vi "Main.vi"() -> ()   [LabVIEW 2019]
uses:
  Sub VIs/State Estimator/Measurements.ctl
  Sub VIs/IMU/IMU Data.ctl
  Sub VIs/Steering Motor Encoder/Steering Motor Encoder Data.ctl
  Sub VIs/GNSS/GNSS Data.ctl
  Sub VIs/State Estimator/State Estimate.ctl
  Sub VIs/Logging/Controller Data.ctl
  Sub VIs/Drive Motor/Drive Motor Data.ctl
  Sub VIs/Steering Motor/Steering Motor Data.ctl
  Sub VIs/Logging/Log Level.ctl
  <vilib>/Platform/TimedLoop/XDataNode/timing_clust.ctl
  <vilib>/Platform/TimedLoop/XDataNode/nitl_modes.ctl
  <vilib>/Platform/TimedLoop/XDataNode/wakeup.ctl
  <vilib>/platform/TimedLoop/XDataNode/XDataNode.xnode
  <vilib>/Platform/TimedLoop/XDataNode/XDNodeRunTimeDep.lvlib
panel:
  out "Motor Controllers (Debug)":T1
  in  "Angular Speed (rad/s)":dbl
  in  "Enable Steering Motor":bool
  out "Steering Motor Enabled":bool
  out "State Estimate (Debug)":T4
  out "Measurements (Debug)":T5
  out "Abort":bool
  in  "Reset Counter":bool
  in  "Stop Button":bool
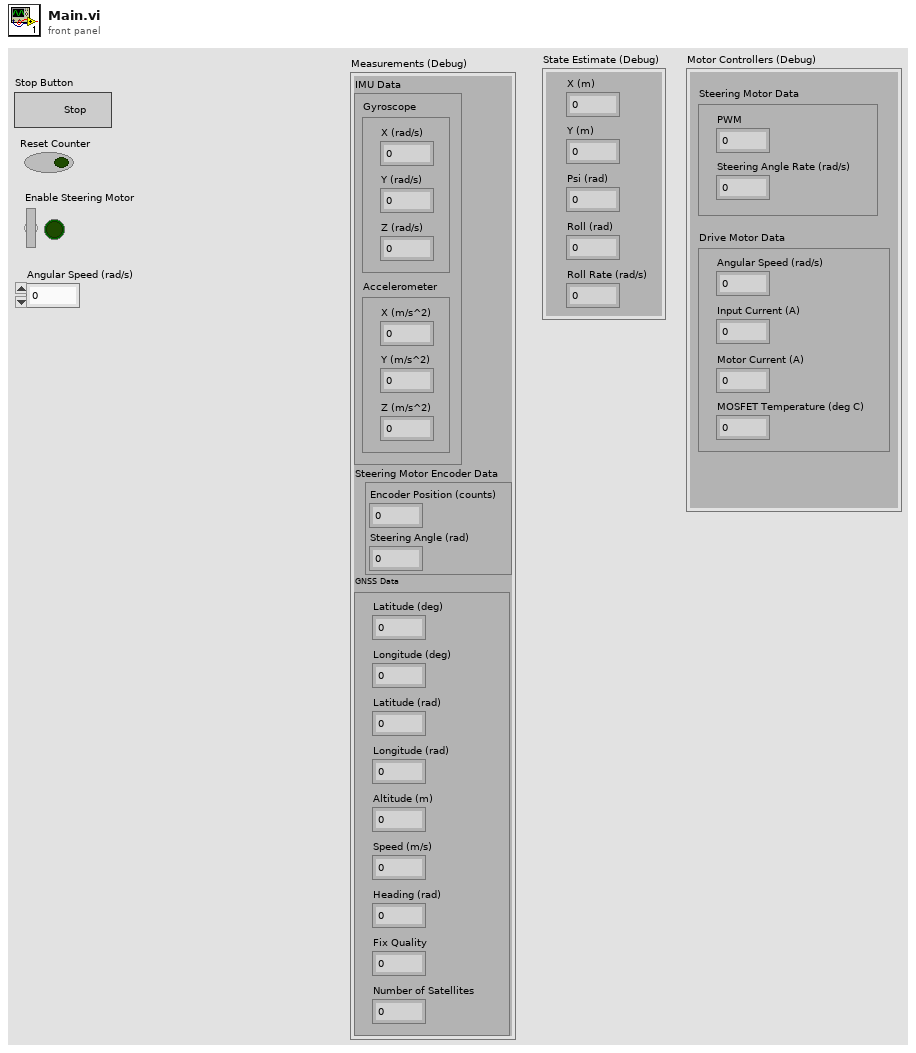
[diagram p1: front panel]
types:
  T1 = typedef "Controller Data.ctl" = cluster{"Drive Motor Data":T2, "Steering Motor Data":T3}
  T2 = typedef "Drive Motor Data.ctl" = cluster{"Angular Speed (rad/s)":dbl, "Input Current (A)":dbl, "Motor Current (A)":dbl, "MOSFET Temperature (deg C)":dbl}
  T3 = typedef "Steering Motor Data.ctl" = cluster{"PWM":dbl, "Steering Angle Rate (rad/s)":dbl}
  T4 = typedef "State Estimate.ctl" = cluster{"X (m)":dbl, "Y (m)":dbl, "Psi (rad)":dbl, "Roll (rad)":dbl, "Roll Rate (rad/s)":dbl}
  T5 = typedef "Measurements.ctl" = cluster{"IMU Data":T6, "Steering Motor Encoder Data":T7, "GNSS Data":T8}
  T6 = typedef "IMU Data.ctl" = cluster{"Gyroscope":cluster{"X (rad/s)":dbl, "Y (rad/s)":dbl, "Z (rad/s)":dbl}, "Accelerometer":cluster{"X (m/s^2)":dbl, "Y (m/s^2)":dbl, "Z (m/s^2)":dbl}}
  T7 = typedef "Steering Motor Encoder Data.ctl" = cluster{"Encoder Position (counts)":i32, "Steering Angle (rad)":dbl}
  T8 = typedef "GNSS Data.ctl" = cluster{"Latitude (rad)":dbl, "Longitude (rad)":dbl, "Altitude (m)":dbl, "Speed (m/s)":dbl, "Heading (rad)":dbl, "Fix Quality":i32, "Number of Satellites":i32, "Latitude (deg)":dbl, "Longitude (deg)":dbl}
  T9 = typedef "XDNodeRunTimeDep.lvlib/timing_clust.ctl" = cluster{"Expected End [f-1]":u64, "Actual End [f-1]":u64, "Finished Late? [f-1]":bool, "Expected End [i-1]":u64, "Actual End [i-1]":u64, "Finished Late? [i-1]":bool, "Expected Start [i]":u64, "Actual Start [i]":u64, "Expected Start [f]":u64, "Actual Start [f]":u64, "Source Name":string, "Structure Name":string, "Period":i64, "Deadline":i64, "Offset":i64, "Start":i64, "Priority":i32, "Timeout":i32, "Mode":T10, "Wakeup Reason":T11, "Error":errorcluster, "Source Type":string, "Secondary Source Type":string, "Global End Time":u64, "Global Start Time":u64, "Frame Duration":u64, "Iteration Duration":u64, "Assigned CPU":i32, "I/O Scan Engine Mode":u32}
  T10 = typedef "XDNodeRunTimeDep.lvlib/nitl_modes.ctl" = enum32{"No Change", "Process missed periods, maintain original phase", "Discard missed periods, maintain original phase", "Process missed periods, ignore original phase", "Discard missed periods, ignore original phase"}
  T11 = typedef "XDNodeRunTimeDep.lvlib/wakeup.ctl" = enum32{"Normal", "Aborted", "Asynchronous wakeup", "Timing source error", "Timed loop error", "Timeout"}
  T12 = typedef "Log Level.ctl" = enum16{"Error", "Warning", "Info"}
  T13 = typedef "Configuration.ctl" = cluster{"Accelerometer Bias":cluster{"X (m/s)":dbl, "Y (m/s)":dbl, "Z (m/s)":dbl}, "Gyroscope Bias":cluster{"X (m/s)":dbl, "Y (m/s)":dbl, "Z (m/s)":dbl}, "Steering Motor Gear Ratio":dbl, "Steering Pully Gear Ratio":dbl, "Steering Encoder CPR":dbl, "Steering Motor Max RPM":dbl, "Wheelbase (m)":dbl, "Fork Angle (rad)":dbl, "Balancing Controller":cluster{"Kp (/s)":dbl, "Kd (1)":dbl}, "Max Allowed Steering Angle (rad)":dbl, "Task Periods":cluster{"Emergency Stop (us)":i64, "IMU (us)":i64, "Steering Motor Encoder (us)":i64, "State Estimator (us)":i64, "Balancing Controller (us)":i64, "GNSS (us)":i64, "Logging (us)":i64, "Drive Motor (us)":i64}, "Drive Motor Gear Ratio":dbl, "Drive Motor UART Delay (ms)":i64}
  T14 = typedef "IMU Handle.ctl" = cluster{"I2C address":u8}
  T15 = typedef "GNSS Handle.ctl" = cluster{"VISA Resource Name":refnum<visa-resource-name>}
  T16 = typedef "Drive Motor Handle.ctl" = cluster{"VISA Resource Name":refnum<visa-resource-name>}
  T17 = typedef "Steering Motor Handle.ctl" = cluster{"Dummy":dbl}
  T18 = typedef "Log Handle.ctl" = cluster{"Data File":refnum<file>, "Event File":refnum<file>}
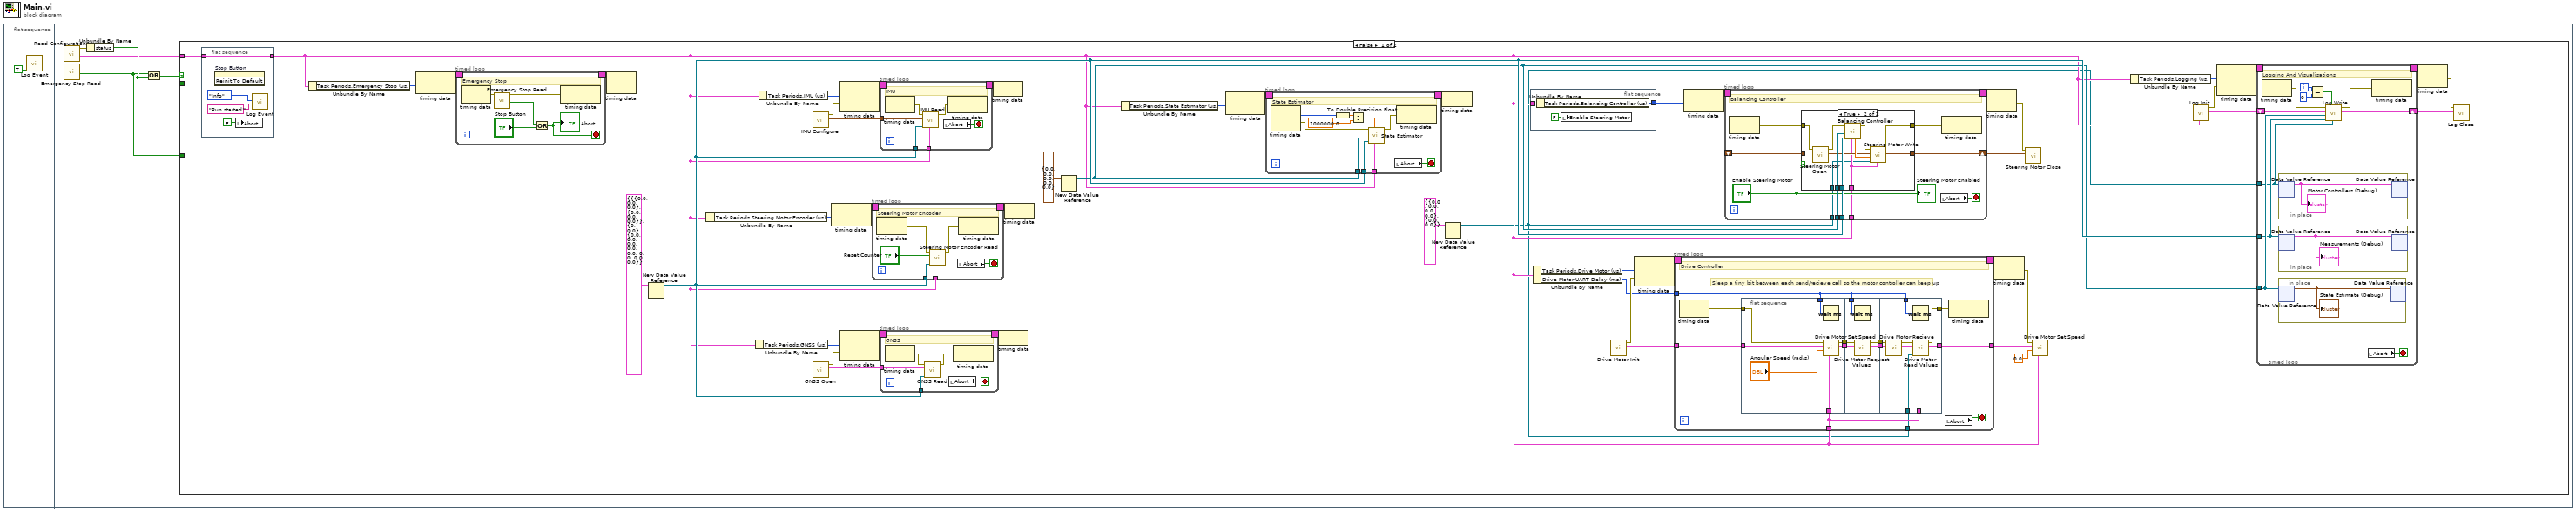
[diagram p0: block diagram]
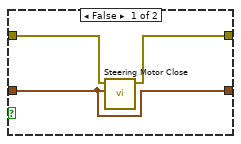
[diagram p2: hidden frame]
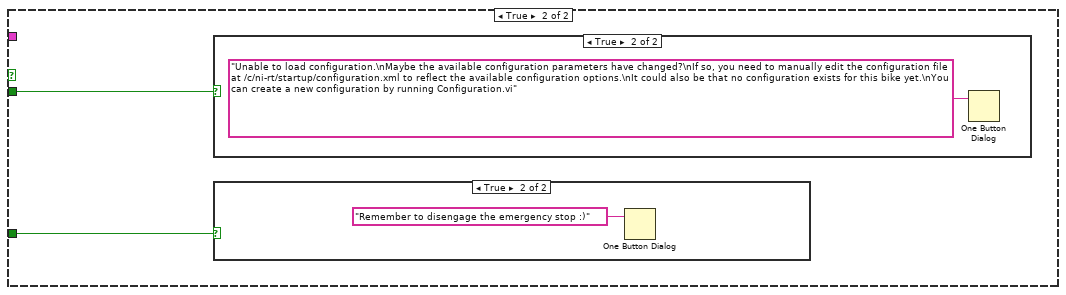
[diagram p3: hidden frame]
diagram:
  n1 = flat-sequence {
    frame #0 {
      n2 = call "Log Event.vi"("Clear Log"=TRUE) -> ()  [unwired: 10 in, 1 out]
    }
    frame #1 {
      n3 = call "Read Configuration.vi"() -> ("Configuration"=w3:T13, "Error Out"=w2:errorcluster)  [unwired: 10 in]
      n4 = call "Emergency Stop Read.vi"() -> ("Emergency Stop"=w4:bool)  [unwired: 10 in, 1 out]
      n5 = Unbundle By Name(w2) -> ("status"=w5:bool)
      n6 = Compound Arithmetic op=OR(w4, w5) -> (w6:bool)
      n7 = case shown="False" w6 {
        tunnel: w5 -> [_ w244]
        tunnel: w4 -> [_ w245]
        tunnel: w3 -> [w26 _]
        frame False {
          n8 = flat-sequence {
            tunnel: [w240] -> w25
            tunnel: w26 -> [w240]
            frame #0 {
              n9 = invoke on="Stop Button" class="Bool (strict)" method="Reinit To Default"() -> ()  [unwired: 3 in, 3 out]
              n10 = local write "Abort"(FALSE ("Abort")) -> ()
              n11 = call "Log Event.vi"("Message"="Run started!", "Log Level"=Log_Level."Info") -> ()  [unwired: 9 in, 1 out]
            }
          }
          n12 = Unbundle By Name(w25) -> ("Task Periods.Emergency Stop (us)"=w50:i64)
          n13 = node-c288(w50) -> (w49:T9)
          n14 = timed-loop {
            timing: w49 -> [_]
            timing-out: [_] -> w48
            stop <- w226 stop-if-true
            # "Emergency Stop"
            n15 = node-c288() -> (w230:errorcluster)  [unwired: 1 in]
            n16 = call "Emergency Stop Read.vi"("Error In"=w230) -> ("Emergency Stop"=w228:bool, "Error Out"=w229:errorcluster)  [unwired: 9 in]
            n17 = Or(x=w228, y="Stop Button") -> (x .or. y?=w226:bool)
            "Abort" <- w226
            n18 = node-c288(w229) -> ()  [unwired: 1 out]
          }
          n19 = node-c288(w48) -> ()  [unwired: 1 out]
          n20 = New Data Value Reference(data value=T5 {"IMU Data"={"Gyroscope"={"X (rad/s)"=0.0, "Y (rad/s)"=0.0, "Z (rad/s)"=0.0}, "Accelerometer"={"X (m/s^2)"=0.0, "Y (m/s^2)"=0.0, "Z (m/s^2)"=0.0}}, "Steering Motor Encoder Data"={"Encoder Position (counts)"=0, "Steering Angle (rad)"=0.0}, "GNSS Data"={"Latitude (rad)"=0.0, "Longitude (rad)"=0.0, "Altitude (m)"=0.0, "Speed (m/s)"=0.0, "Heading (rad)"=0.0, "Fix Quality"=0, "Number of Satellites"=0, "Latitude (deg)"=0.0, "Longitude (deg)"=0.0}} ("Cluster")) -> (data value reference=w52:refnum<data-value>)  [unwired: 1 in, 1 out]
          n21 = Unbundle By Name(w25) -> ("Task Periods.Steering Motor Encoder (us)"=w34:i64)
          n22 = Unbundle By Name(w25) -> ("Task Periods.GNSS (us)"=w31:i64)
          n23 = Unbundle By Name(w25) -> ("Task Periods.IMU (us)"=w35:i64)
          n24 = call "IMU Configure.vi"() -> ("IMU Handle"=w36:T14, "Error Out"=w37:errorcluster)  [unwired: 10 in]
          n25 = call "GNSS Open.vi"() -> ("GNSS Handle"=w32:T15, "Error Out"=w33:errorcluster)  [unwired: 10 in]
          n26 = node-c288(w34) -> (w41:T9)
          n27 = node-c288(w35, w37) -> (w43:T9)
          n28 = node-c288(w31, w33) -> (w39:T9)
          n29 = timed-loop {
            timing: w41 -> [_]
            timing-out: [_] -> w40
            tunnel: w52 -> [w159]
            tunnel: w25 -> [_]
            stop <- w160 stop-if-true
            # "Steering Motor Encoder"
            n30 = node-c288() -> (w163:errorcluster)  [unwired: 1 in]
            n31 = call "Steering Motor Encoder Read.vi"("Measurement In"=w159, "Reset Counter"="Reset Counter", "Error In"=w163) -> ("Error Out"=w162:errorcluster)  [unwired: 6 in, 2 out]
            n32 = local read "Abort"() -> (w160:bool)
            n33 = node-c288(w162) -> ()  [unwired: 1 out]
          }
          n34 = timed-loop {
            timing: w43 -> [_]
            timing-out: [_] -> w42
            tunnel: w36 -> [w176]
            tunnel: w52 -> [w174]
            tunnel: w25 -> [w173]
            stop <- w175 stop-if-true
            # "IMU"
            n35 = node-c288() -> (w178:errorcluster)  [unwired: 1 in]
            n36 = call "IMU Read.vi"("Configuration"=w173, "Measurement In"=w174, "IMU Handle"=w176, "Error In"=w178) -> ("Error Out"=w177:errorcluster)  [unwired: 5 in, 2 out]
            n37 = local read "Abort"() -> (w175:bool)
            n38 = node-c288(w177) -> ()  [unwired: 1 out]
          }
          n39 = timed-loop {
            timing: w39 -> [_]
            timing-out: [_] -> w38
            tunnel: w32 -> [w148]
            tunnel: w52 -> [w144]
            stop <- w145 stop-if-true
            # "GNSS"
            n40 = node-c288() -> (w147:errorcluster)  [unwired: 1 in]
            n41 = call "GNSS Read.vi"("Measurement In"=w144, "GNSS Handle"=w148, "Error In"=w147) -> ("Error Out"=w146:errorcluster)  [unwired: 6 in, 2 out]
            n42 = local read "Abort"() -> (w145:bool)
            n43 = node-c288(w146) -> ()  [unwired: 1 out]
          }
          n44 = node-c288(w42) -> ()
          n45 = node-c288(w38) -> ()
          n46 = node-c288(w40) -> ()
          n47 = New Data Value Reference(data value=T4 {"X (m)"=0.0, "Y (m)"=0.0, "Psi (rad)"=0.0, "Roll (rad)"=0.0, "Roll Rate (rad/s)"=0.0} ("State Estimate")) -> (data value reference=w51:refnum<data-value>)  [unwired: 1 in, 1 out]
          n48 = Unbundle By Name(w25) -> ("Task Periods.State Estimator (us)"=w28:i64)
          n49 = node-c288(w28) -> (w30:T9)
          n50 = timed-loop {
            timing: w30 -> [_]
            timing-out: [_] -> w29
            tunnel: w52 -> [w126]
            tunnel: w51 -> [w125]
            tunnel: w25 -> [w124]
            stop <- w133 stop-if-true
            # "State Estimator"
            n51 = node-c288() -> (w130:i64, w132:errorcluster)  [unwired: 1 in]
            n52 = To Double Precision Float(number=w130) -> (double precision float=w129:dbl)
            n53 = Divide(x=w129, y=1000000.0) -> (x/y=w127:dbl)
            n54 = call "State Estimator.vi"("Configuration"=w124, "Ts"=w127, "Measurement In"=w126, "State Estimate In"=w125, "Error In"=w132) -> ("Error out"=w131:errorcluster)  [unwired: 4 in, 2 out]
            n55 = local read "Abort"() -> (w133:bool)
            n56 = node-c288(w131) -> ()  [unwired: 1 out]
          }
          n57 = node-c288(w29) -> ()
          n58 = New Data Value Reference(data value=T1 {"Drive Motor Data"={"Angular Speed (rad/s)"=0.0, "Input Current (A)"=0.0, "Motor Current (A)"=0.0, "MOSFET Temperature (deg C)"=0.0}, "Steering Motor Data"={"PWM"=0.0, "Steering Angle Rate (rad/s)"=0.0}}) -> (data value reference=w23:refnum<data-value>)  [unwired: 1 in, 1 out]
          n59 = flat-sequence {
            tunnel: [w190] -> w27
            tunnel: w25 -> [w189]
            frame #0 {
              n60 = Unbundle By Name(w189) -> ("Task Periods.Balancing Controller (us)"=w190:i64)
              n61 = local write "Enable Steering Motor"(FALSE ("Enable Steering Motor")) -> ()
            }
          }
          n62 = Unbundle By Name(w25) -> ("Task Periods.Drive Motor (us)"=w20:i64, "Drive Motor UART Delay (ms)"=w7:i64)
          n63 = call "Drive Motor Init.vi"() -> ("Drive Motor Handle"=w18:T16, "Error Out"=w17:errorcluster)  [unwired: 10 in]
          n64 = node-c288(w20, w17) -> (w22:T9)
          n65 = timed-loop {
            timing: w22 -> [_]
            timing-out: [_] -> w21
            tunnel: w18 -> [w88]
            tunnel: [w87] -> w16
            tunnel: w25 -> [w86]
            tunnel: w23 -> [w85]
            tunnel: w7 -> [w80]
            stop <- w91 stop-if-true
            # "Sleep a tiny bit between each send/recieve call so the motor controller can keep up"
            # "Drive Controller"
            n66 = node-c288() -> (w89:errorcluster)  [unwired: 1 in]
            n67 = flat-sequence {
              tunnel: [w98] -> w84
              tunnel: w89 -> [w97]
              tunnel: w88 -> [w96]
              tunnel: [w95] -> w83
              tunnel: w86 -> [w93]
              tunnel: w80 -> [w92]
              tunnel: [w103] -> w82
              tunnel: w84 -> [w102]
              tunnel: w83 -> [w101]
              tunnel: [w100] -> w81
              tunnel: w80 -> [w99]
              tunnel: w82 -> [w112]
              tunnel: [w111] -> w90
              tunnel: w81 -> [w110]
              tunnel: [w109] -> w87
              tunnel: w86 -> [w108]
              tunnel: w80 -> [w107]
              tunnel: w85 -> [w106]
              frame #0 {
                n68 = Wait (ms)(milliseconds to wait=w92) -> ()  [unwired: 1 out]
                n69 = call "Drive Motor Set Speed.vi"("Configuration"=w93, "Angular Speed (rad/s)"="Angular Speed (rad/s)", "Drive Motor Handle In"=w96, "Error In"=w97) -> ("Drive Motor Handle Out"=w95:T16, "Error Out"=w98:errorcluster)  [unwired: 6 in]
              }
              frame #1 {
                n70 = Wait (ms)(milliseconds to wait=w99) -> ()  [unwired: 1 out]
                n71 = call "Drive Motor Request Values.vi"("Drive Motor Handle In"=w101, "Error In"=w102) -> ("Drive Motor Handle Out"=w100:T16, "Error Out"=w103:errorcluster)  [unwired: 8 in]
              }
              frame #2 {
                n72 = call "Drive Motor Recieve.vi"("Drive Motor Handle In"=w110, "Error In"=w112) -> ("Drive Motor Handle Out"=w104:T16, "Error Out"=w105:errorcluster)  [unwired: 8 in]
                n73 = Wait (ms)(milliseconds to wait=w107) -> ()  [unwired: 1 out]
                n74 = call "Drive Motor Read Values.vi"("Configuration"=w108, "Controller Data In"=w106, "Drive Motor Handle In"=w104, "Error In"=w105) -> ("Drive Motor Handle Out"=w109:T16, "Error Out"=w111:errorcluster)  [unwired: 4 in, 2 out]
              }
            }
            n75 = local read "Abort"() -> (w91:bool)
            n76 = node-c288(w90) -> ()  [unwired: 1 out]
          }
          n77 = node-c288(w27) -> (w47:T9)
          n78 = timed-loop {
            timing: w47 -> [_]
            timing-out: [_] -> w46
            tunnel: w51 -> [w197]
            tunnel: w52 -> [w196]
            shift-right: [w198] -> w45
            shift-left: _ -> [w194]
            tunnel: w25 -> [w193]
            tunnel: w23 -> [w192]
            stop <- w201 stop-if-true
            # "Balancing Controller"
            n79 = node-c288() -> (w200:errorcluster)  [unwired: 1 in]
            n80 = case shown="True" "Enable Steering Motor" {
              tunnel: w200 -> [w204 w209]
              tunnel: [w203 w214] -> w199
              tunnel: [w202 w213] -> w198
              tunnel: w197 -> [_ w211]
              tunnel: w196 -> [_ w210]
              tunnel: w194 -> [w202 _]
              tunnel: w193 -> [_ w206]
              tunnel: w192 -> [_ w205]
              frame False {
                n81 = call "Steering Motor Close.vi"("Steering Motor Handle"=w202, "Error In"=w204) -> ("Error Out"=w203:errorcluster)  [unwired: 9 in]
              }
              frame True {
                n82 = call "Steering Motor Open.vi"("Error In"=w209) -> ("Steering Motor Handle"=w207:T17, "Error Out"=w208:errorcluster)  [unwired: 9 in]
                n83 = call "Balancing Controller.vi"("Configuration"=w206, "Measurement In"=w210, "State Estimate In"=w211, "Error In"=w208) -> ("Error Out"=w215:errorcluster, "Steering Angle Rate (rad/s)"=w212:dbl)  [unwired: 4 in, 2 out]
                n84 = call "Steering Motor Write.vi"("Configuration"=w206, "Controller Data In"=w205, "Steering Angle Rate (rad/s)"=w212, "Steering Motor Handle In"=w207, "Error In"=w215) -> ("Steering Motor Handle Out"=w213:T17, "Error Out"=w214:errorcluster)  [unwired: 3 in, 2 out]
              }
            }
            n85 = local read "Abort"() -> (w201:bool)
            n86 = node-c288(w199) -> ()  [unwired: 1 out]
            "Steering Motor Enabled" <- "Enable Steering Motor"
          }
          n87 = node-c288(w46) -> (w44:errorcluster)
          n88 = node-c288(w21) -> (w19:errorcluster)
          n89 = call "Steering Motor Close.vi"("Steering Motor Handle"=w45, "Error In"=w44) -> ()  [unwired: 9 in, 1 out]
          n90 = call "Drive Motor Set Speed.vi"("Configuration"=w25, "Angular Speed (rad/s)"=0.0, "Drive Motor Handle In"=w16, "Error In"=w19) -> ()  [unwired: 6 in, 2 out]
          n91 = Unbundle By Name(w25) -> ("Task Periods.Logging (us)"=w12:i64)
          n92 = call "Log Init.vi"("Configuration"=w25) -> ("Log Handle"=w8:T18, "Error Out"=w11:errorcluster)  [unwired: 9 in]
          n93 = node-c288(w12, w11) -> (w14:T9)
          n94 = timed-loop {
            timing: w14 -> [_]
            timing-out: [_] -> w13
            tunnel: w52 -> [w60]
            tunnel: w51 -> [w61]
            shift-right: [w62] -> w9
            shift-left: w8 -> [w57]
            tunnel: w23 -> [w55]
            i -> [w59]
            stop <- w65 stop-if-true
            # "Logging And Visualisations"
            n95 = node-c288() -> (w64:errorcluster)  [unwired: 1 in]
            n96 = in-place {
              n97 = in-place-dvr #1(w55) -> (w66:T1)  [unwired: 1 out]
              "Motor Controllers (Debug)" <- w66
              n98 = in-place-dvr #1(w66) -> ()  [unwired: 2 out]
            }
            n99 = in-place {
              n100 = in-place-dvr #2(w60) -> (w68:T5)  [unwired: 1 out]
              "Measurements (Debug)" <- w68
              n101 = in-place-dvr #2(w68) -> ()  [unwired: 2 out]
            }
            n102 = in-place {
              n103 = in-place-dvr #3(w61) -> (w67:T4)  [unwired: 1 out]
              "State Estimate (Debug)" <- w67
              n104 = in-place-dvr #3(w67) -> ()  [unwired: 2 out]
            }
            n105 = Equal?(x=w59, y=0) -> (x = y?=w56:bool)
            n106 = call "Log Write.vi"("Controller Data In"=w55, "Write Header"=w56, "Measurement In"=w60, "State Estimate In"=w61, "Log Handle In"=w57, "Error In"=w64) -> ("Log Handle Out"=w62:T18, "Error Out"=w63:errorcluster)  [unwired: 4 out]
            n107 = local read "Abort"() -> (w65:bool)
            n108 = node-c288(w63) -> ()  [unwired: 1 out]
          }
          n109 = node-c288(w13) -> (w10:errorcluster)
          n110 = call "Log Close.vi"("Log Handle In"=w9, "Error In"=w10) -> ()  [unwired: 9 in, 1 out]
        }
        frame True {
          n111 = case shown="True" w244 {
            frame False {
            }
            frame True {
              n112 = One Button Dialog(message="Unable to load configuration.\nMaybe the available configuration parameters have changed?\nIf so, you need to manually edit the configuration file at /c/ni-rt/startup/configuration.xml to reflect the available configuration options.\nIt could also be that no configuration exists for this bike yet.\nYou can create a new configuration by running Configuration.vi") -> ()  [unwired: 1 in, 1 out]
            }
          }
          n113 = case shown="True" w245 {
            frame False {
            }
            frame True {
              n114 = One Button Dialog(message="Remember to disengage the emergency stop :)") -> ()  [unwired: 1 in, 1 out]
            }
          }
        }
      }
    }
  }
